vi "Main.vi"(8 "error in (no error)":errorcluster, 11 "GalvoBase in":refnum<class "InVivo_ImagingModeSPIM.lvclass">) -> (0 "error out":errorcluster, 3 "component":refnum<class "InVivo_ImagingModeSPIM.lvclass">)   [LabVIEW 2012, in "InVivo_ImagingModeSPIM.lvclass"]
doc: "Main VI of the component."
uses:
  InVivo_ImagingModeSPIM.lvclass
  <vilib>/Distrio/LabbitMQ/Connection/Connection.lvclass
  <vilib>/Distrio/LabbitMQ/Exchange/Exchange.lvclass
  <vilib>/Distrio/LabbitMQ/Queue/Queue.lvclass
  <vilib>/Distrio/Murmex/TerminateMessage/TerminateMessage.lvclass
  Controls/waveform_enum.ctl
  Control 4.ctl
  InVivo_ImagingModeSPIM.lvclass/InVivo_ImagingModeSPIM.ctl
  <vilib>/Distrio/Murmex/InitialiseMessage/InitialiseMessage.lvclass
  <vilib>/Distrio/Murmex/ConfigureMessage/ConfigureMessage.lvclass
  <vilib>/Distrio/Murmex/StopMessage/StopMessage.lvclass
  <vilib>/Distrio/Murmex/StartMessage/run mode enum.ctl
  <vilib>/Distrio/Murmex/StartMessage/StartMessage.lvclass
  <vilib>/Distrio/Murmex/Murmex/update_cluster.ctl
  <vilib>/Distrio/Murmex/Murmex/Set configure at initialise.vi
  <vilib>/Distrio/Murmex/Murmex/Set VI reference.vi
  <vilib>/Distrio/Murmex/Murmex/Get ID.vi
  <vilib>/Distrio/Murmex/Murmex/Set relay start stop to observers.vi
  <vilib>/Distrio/Murmex/Murmex/Set log reference.vi
  <vilib>/Distrio/Murmex/Murmex/Set license required.vi
  <vilib>/Distrio/Murmex/StartMessage/Set run mode.vi
  <vilib>/Distrio/Murmex/Murmex/Murmex.lvclass
panel:
  in  "button::quit":bool
  in  "button:start_finite":bool
  in  "button:start_free-run":bool
  in  "button::configure":bool
  in  "Tab Control":T1(tab)=enum."Camera"
  in  "Phase 3":dbl[unit] caption="phase" min=-6.283185307179586 max=6.283185307179586 step=0.0017453292519943296
  in  "Offset 3":dbl[unit] caption="offset" min=-5.0 max=5.0 step=0.01
  in  "Amplitude 3":dbl[unit] caption="amplitude" min=0.0 max=5.0 step=0.01
  in  "Phase 2":dbl[unit]=3.14159 caption="phase" min=-6.283185307179586 max=6.283185307179586 step=0.0017453292519943296
  in  "Offset 2":dbl[unit] caption="offset" min=-5.0 max=5.0 step=0.01
  in  "Amplitude 2":dbl[unit] caption="amplitude" min=0.0 max=5.0 step=0.01
  in  "Phase 1":dbl[unit]=3.14159 caption="phase" min=-6.283185307179586 max=6.283185307179586 step=0.0017453292519943296
  in  "shape":T2=enum."sawtooth"
  in  "Offset 1":dbl[unit] caption="offset" min=-5.0 max=5.0 step=0.01
  in  "Amplitude 1":dbl[unit] caption="amplitude" min=0.0 max=5.0 step=0.01
  in  "Amplitude 4":dbl[unit] caption="amplitude" min=0.0 max=5.0 step=0.01
  in  "Offset 4":dbl[unit] caption="offset" min=-5.0 max=5.0 step=0.01
  in  "Phase 4":dbl[unit] caption="phase" min=-6.283185307179586 max=6.283185307179586 step=0.0017453292519943296
  in  "AOTFwaveform":T3
  in  "frame time":dbl[unit]=1.0
  in  "HSYNC pulses":dbl=2048.0 format="%#_6f"
  in  "digital ratio":dbl(knob)=0.5 min=0.0 max=1.0 step=0.02 scale=0.0..1.0
  in  "pulses per pixel":i32 min=0 max=20 step=2
  out "log":string="\r\n16:45:19.783 24/11/2014: initialise from SPIM to SPIM\r\n16:45:20.308 24/11/2014: inform from DAQmxIO to SPIM\r\n16:45:20.427 24/11/2014: inform from SPIM to SPIM\r\n16:45:20.475 24/11/2014: update from SPIM to SPIM\r\n16:45:20.579 24/11/2014: inspect from SPIM to SPIM\r\n16:45:20.660 24/11/2014: inform from SPIM to SPIM\r\n16:45:23.740 24/11/2014: update from SPIM to SPIM\r\n16:45:23.747 24/11/2014: inspect from SPIM to SPIM\r\n16:45:23.824 24/11/2014: inform from SPIM to SPIM\r\n16:45:23.956 24/11/2014: update from SPIM to SPIM\r\n16:45:23.962 24/11/2014: inspect from SPIM to SPIM\r\n16:45:24.038 24/11/2014: inform from SPIM to SPIM\r\n16:45:25.804 24/11/2014: update from SPIM to SPIM\r\n16:45:25.810 24/11/2014: inspect from SPIM to SPIM\r\n16:45:25.891 24/11/2014: inform from SPIM to SPIM\r\n16:45:26.005 24/11/2014: update from SPIM to SPIM\r\n16:45:26.012 24/11/2014: inspect from SPIM to SPIM\r\n16:45:26.088 24/11/2014: inform from SPIM to SPIM\r\n16:45:26.428 24/11/2014: update from SPIM to SPIM\r\n16:45:26.434 24/11/2014: inspect from SPIM to SPIM\r\n16:45:26.514 24/11/2014: inform from SPIM to SPIM\r\n16:45:26.620 24/11/2014: update from SPIM to SPIM\r\n16:45:26.626 24/11/2014: inspect from SPIM to SPIM\r\n16:45:26.703 24/11/2014: inform from SPIM to SPIM\r\n16:45:27.100 24/11/2014: update from SPIM to SPIM\r\n16:45:27.108 24/11/2014: inspect from SPIM to SPIM\r\n16:45:27.184 24/11/2014: inform from SPIM to SPIM\r\n16:45:27.292 24/11/2014: update from SPIM to SPIM\r\n16:45:27.298 24/11/2014: inspect from SPIM to SPIM\r\n16:45:27.380 24/11/2014: inform from SPIM to SPIM\r\n16:45:27.660 24/11/2014: update from SPIM to SPIM\r\n16:45:27.666 24/11/2014: inspect from SPIM to SPIM\r\n16:45:27.743 24/11/2014: inform from SPIM to SPIM\r\n16:45:27.852 24/11/2014: update from SPIM to SPIM\r\n16:45:27.858 24/11/2014: inspect from SPIM to SPIM\r\n16:45:27.934 24/11/2014: inform from SPIM to SPIM\r\n16:45:28.332 24/11/2014: update from SPIM to SPIM\r\n16:45:28.338 24/11/2014: inspect from SPIM to SPIM\r\n16:45:28.421 24/11/2014: inform from SPIM to SPIM\r\n16:45:30.144 24/11/2014: update from SPIM to SPIM\r\n16:45:30.150 24/11/2014: inspect from SPIM to SPIM\r\n16:45:30.232 24/11/2014: inform from SPIM to SPIM\r\n16:45:34.417 24/11/2014: terminate from SPIM to SPIM"
  in  "ID":string="SPIM"
  out "terminate?":bool=TRUE
  # "galvo 1"
  # "galvo 2"
  # "galvo 3"
  # "AOTF"
  # "ImagingModeSPIM\n\nDeveloped by:\n\nMarcel van 't Hoff PhD, \nMarie Caroline Muellenbroich PhD, \nLudovico Silvestri PhD,\n   University of Florence, 2014"
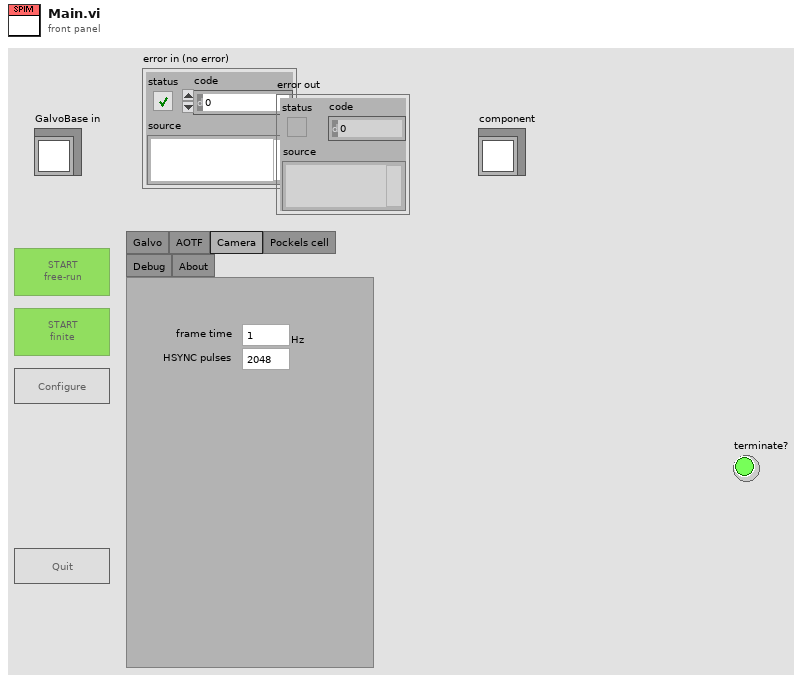
[diagram p1: front panel]
types:
  T1 = enum32{"Galvo", "AOTF", "Camera", "Pockels cell", "Debug", "About"}
  T2 = typedef "InVivo_ImagingModeSPIM.lvclass/waveform_enum.ctl" = enum16{"triangular", "sawtooth", "sinusodial"}
  T3 = typedef "InVivo_ImagingModeSPIM.lvclass/Control 4.ctl" = enum16{"Triangular", "Sawtooth", "Sinusoidal"}
  T4 = enum8{"Enabled", "Disabled", "Disabled and Grayed Out"}
  T5 = typedef "Murmex.lvlib/StartMessage.lvclass/run mode enum.ctl" = enum16{"infinite", "finite"}
  T6 = typedef "Murmex.lvlib/Murmex.lvclass/update_cluster.ctl" = cluster{"target ID":string, "key chains":string[], "values":variant[]}
  T7 = typedef "Murmex.lvlib/Murmex.lvclass/command_enum.ctl" = enum16{"null", "initialise", "reset", "terminate", "acknowledge", "update", "inspect", "inform", "proceed", "start", "stop", "fetch", "configure", "generic"}
  T8 = typedef "Murmex.lvlib/Murmex.lvclass/Event type enumerations.ctl" = enum16{"before", "after"}
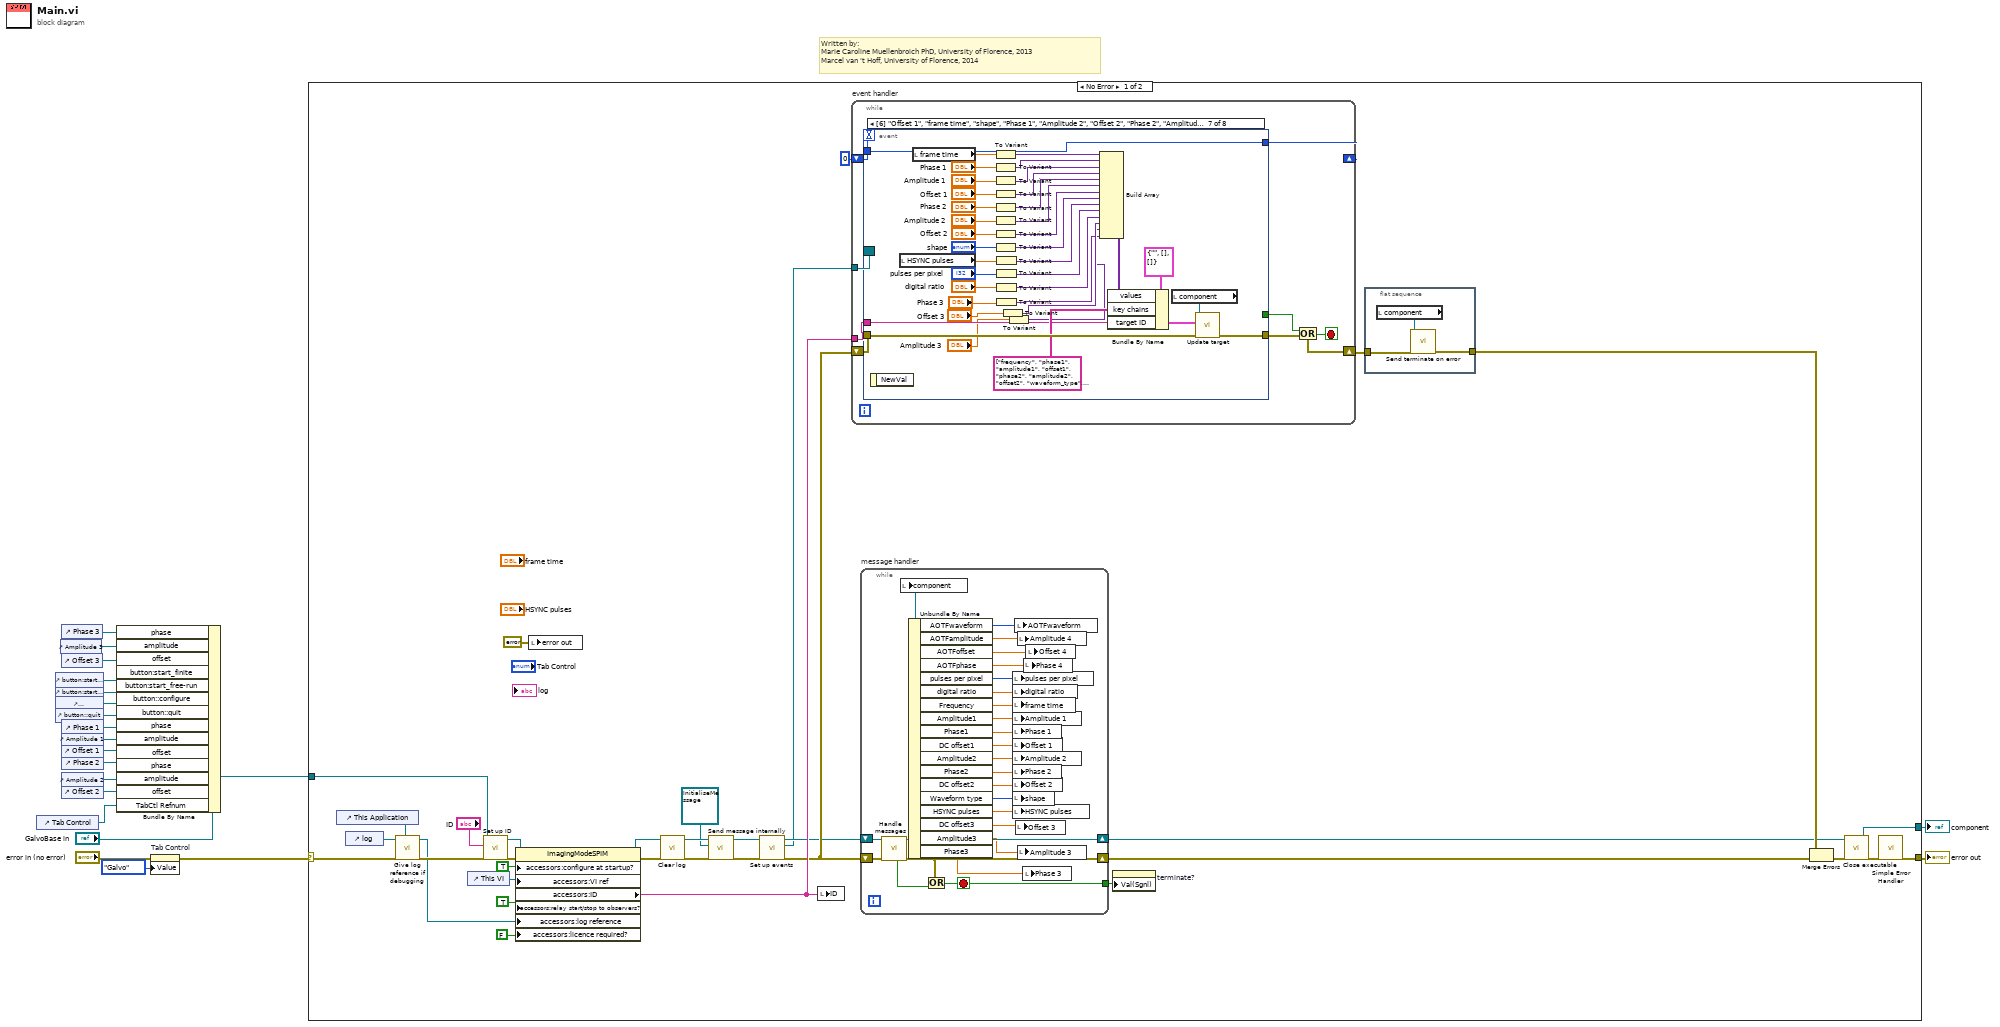
[diagram p0: block diagram]
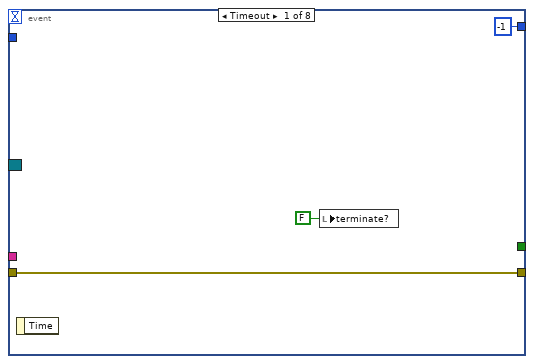
[diagram p2: hidden frame]
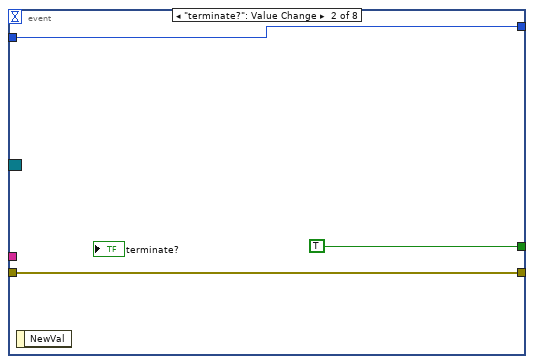
[diagram p3: hidden frame]
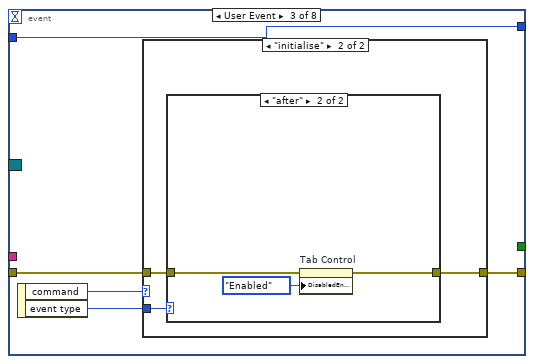
[diagram p4: hidden frame]
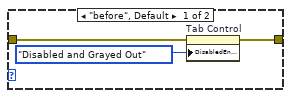
[diagram p6: hidden frame]
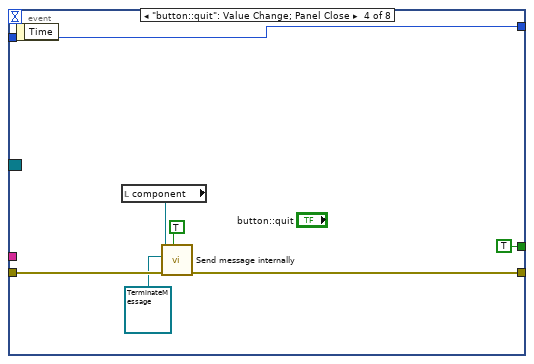
[diagram p7: hidden frame]
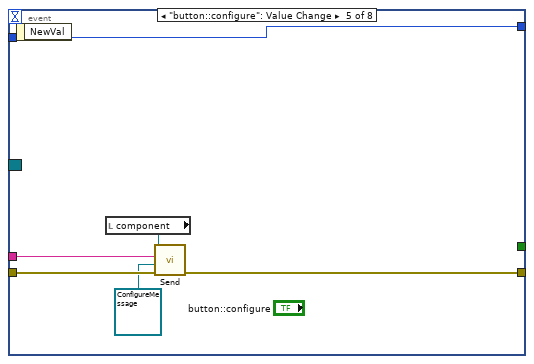
[diagram p8: hidden frame]
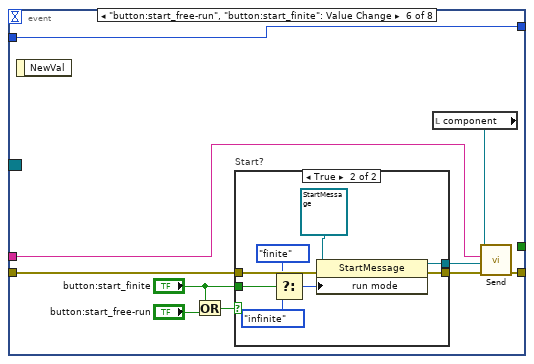
[diagram p9: hidden frame]
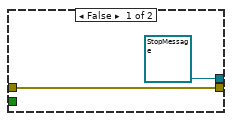
[diagram p10: hidden frame]
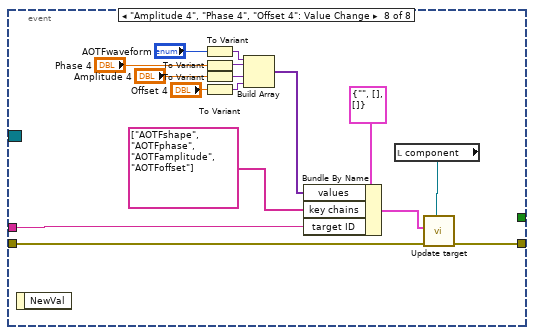
[diagram p11: hidden frame]
diagram:
  # "Written by:\nMarie Caroline Muellenbroich PhD, University of Florence, 2013 \nMarcel van 't Hoff, University of Florence, 2014"
  n1 = control-ref of="Tab Control"() -> (w1:refnum<vi>)
  n2 = control-ref of="button:start_finite"() -> (w18:refnum<vi>)
  n3 = control-ref of="button:start_free-run"() -> (w15:refnum<vi>)
  n4 = control-ref of="button::configure"() -> (w16:refnum<vi>)
  n5 = control-ref of="button::quit"() -> (w17:refnum<vi>)
  n6 = control-ref of="Amplitude 3"() -> (w4:refnum<vi>)
  n7 = control-ref of="Phase 3"() -> (w5:refnum<vi>)
  n8 = control-ref of="Offset 3"() -> (w3:refnum<vi>)
  n9 = control-ref of="Phase 1"() -> (w14:refnum<vi>)
  n10 = control-ref of="Amplitude 1"() -> (w13:refnum<vi>)
  n11 = control-ref of="Offset 1"() -> (w12:refnum<vi>)
  n12 = control-ref of="Phase 2"() -> (w11:refnum<vi>)
  n13 = control-ref of="Amplitude 2"() -> (w10:refnum<vi>)
  n14 = control-ref of="Offset 2"() -> (w9:refnum<vi>)
  n15 = Bundle By Name(cluster="GalvoBase in", "phase"=w5, "amplitude"=w4, "offset"=w3, "button:start_finite"=w18, "button:start_free-run"=w15, "button::configure"=w16, "button::quit"=w17, "phase"=w14, "amplitude"=w13, "offset"=w12, "phase"=w11, "amplitude"=w10, "offset"=w9, "TabCtl Refnum"=w1) -> (w19:refnum<class "InVivo_ImagingModeSPIM.lvclass">)
  n16 = property on="Tab Control" class="TabCtl (strict)"(error in="error in (no error)", "Value"=T1."Galvo" ("Tab Control")) -> (error out=w6:errorcluster)  [unwired: 1 in, 1 out]
  n17 = case shown="No Error" w6 {
    selector: w6 -> [w26 w199]
    tunnel: [w56 w199] -> w21
    tunnel: w19 -> [w38 w200]
    tunnel: [w55 w200] -> w7
    frame No Error {
      n18 = control-ref of="This Application"() -> (w22:refnum<vi>)
      n19 = control-ref of="log"() -> (w24:refnum<vi>)
      n20 = call "Give log reference if debugging.vi"("application ref"=w22, "error in (no error)"=w26, "log reference in"=w24) -> ("error out"=w25:errorcluster, "log reference out"=w23:refnum<vi>)  [unwired: 6 in, 1 out]
      n21 = control-ref of="This VI"() -> (w53:refnum<vi>)
      n22 = call <vilib>:"Set up ID.vi"("error in (no error)"=w25, "component ID"="ID", "MurmexBase in"=w38) -> ("error out"=w50:errorcluster, "MurmexBase out"=w51:refnum<class "InVivo_ImagingModeSPIM.lvclass">)  [unwired: 6 in, 1 out]
      n23 = property class="ImagingModeSPIM"(reference=w51, error in=w50, "accessors:configure at startup?"=TRUE ("configure at startup?"), "accessors:VI ref"=w53, "accessors:relay start/stop to observers?"=TRUE ("relay start/stop to observers?"), "accessors:log reference"=w23, "accessors:licence required?"=FALSE ("licence required?")) -> (reference out=w35:refnum<class "InVivo_ImagingModeSPIM.lvclass">, error out=w37:errorcluster, "accessors:ID"=w40:string)
      n24 = local write "error out"(errorcluster {"status"=FALSE, "code"=0, "source"=""} ("error out")) -> ()
      n25 = call <vilib>:"Clear log.vi"("error in (no error)"=w37, "MurmexBase in"=w35) -> ("error out"=w36:errorcluster, "MurmexBase out"=w34:refnum<class "InVivo_ImagingModeSPIM.lvclass">)  [unwired: 8 in]
      n26 = call <vilib>:"Send message internally.vi"("error in (no error)"=w36, "Message"=refnum<class "InitialiseMessage.lvclass"> refnum ("Murmex.lvlib:InitialiseMessage"), "Murmex in"=w34) -> ("error out"=w31:errorcluster, "Murmex out"=w29:refnum<class "InVivo_ImagingModeSPIM.lvclass">)  [unwired: 7 in]
      n27 = call <vilib>:"Set up events.vi"("error in (no error)"=w31, "MurmexBase in"=w29) -> ("error out"=w30:errorcluster, "Event Registration Refnum"=w27:refnum<event-registration>, "MurmexBase out"=w28:refnum<class "InVivo_ImagingModeSPIM.lvclass">)  [unwired: 7 in]
      n28 = local write "ID"(w40) -> ()
      n29 = while "event handler" {
        shift-right: [w65] -> w48
        shift-left: w30 -> [w67]
        shift-right: [w61] -> _
        shift-left: 0 -> [w62]
        tunnel: w40 -> [w63]
        tunnel: w27 -> [w60]
        stop <- w64 stop-if-true
        n30 = event shown="[6] \"Offset 1\", \"frame time\", \"shape\", \"Phase 1\", \"Amplitude 2\", \"Offset 2\", \"Phase 2\", \"Amplitude 1\", \"HSYNC pulses\", \"pulses per pixel\", \"digital ratio\", \"Offset 3\", \"Phase 3\", \"Amplitude 3\": Value Change" {
          selector: w60 -> [_ _ _ _ _ _ _ _]
          dyn-events: _ -> [_ _ _ _ _ _ _ _]
          timeout: w62 -> [_ _ _ _ _ _ _ _]
          tunnel: [w70 w73 w75 w95 w100 w105 w157 w165] -> w65
          tunnel: w67 -> [w70 w73 w76 w94 w101 w110 w158 w166]
          tunnel: [_ TRUE ("configure at startup?") _ TRUE ("configure at startup?") _ _ _ _] -> w66
          tunnel: w63 -> [_ _ _ _ w99 w102 w136 w170]
          tunnel: w62 -> [_ w71 w74 w92 w98 w111 w144 _]
          tunnel: [-1 w71 w74 w92 w98 w111 w144 _] -> w61
          event Timeout {
            n31 = event-data() -> ()  [unwired: 1 in, 1 out]
            n32 = local write "terminate?"(FALSE ("terminate?")) -> ()
          }
          event "terminate?": Value Change {
            n33 = event-data() -> ()  [unwired: 1 in, 1 out]
          }
          event User Event {
            n34 = event-data() -> ("command"=w78:T7, "event type"=w77:T8)  [unwired: 1 in]
            n35 = case shown="\"initialise\"" w78 {
              tunnel: w77 -> [_ w82]
              tunnel: w76 -> [w79 w81]
              tunnel: [w79 w80] -> w75
              frame "null", Default {
              }
              frame "initialise" {
                n36 = case shown="\"after\"" w82 {
                  tunnel: w81 -> [w85 w88]
                  tunnel: [w84 w87] -> w80
                  frame "before", Default {
                    n37 = property on="Tab Control" class="TabCtl (strict)"(error in=w85, "DisabledEnum"=T4."Disabled and Grayed Out" ("Disabled")) -> (error out=w84:errorcluster)  [unwired: 1 in, 1 out]
                  }
                  frame "after" {
                    n38 = property on="Tab Control" class="TabCtl (strict)"(error in=w88, "DisabledEnum"=T4."Enabled" ("Disabled")) -> (error out=w87:errorcluster)  [unwired: 1 in, 1 out]
                  }
                }
              }
            }
          }
          event "button::quit": Value Change; Panel Close {
            n39 = event-data() -> ()  [unwired: 1 in, 1 out]
            n40 = local read "component"() -> (w91:refnum<class "InVivo_ImagingModeSPIM.lvclass">)
            n41 = call <vilib>:"Send message internally.vi"("priority message? (F)"=TRUE, "error in (no error)"=w94, "Message"=refnum<class "TerminateMessage.lvclass"> refnum ("Murmex.lvlib:TerminateMessage"), "Murmex in"=w91) -> ("error out"=w95:errorcluster)  [unwired: 6 in, 1 out]
          }
          event "button::configure": Value Change {
            n42 = event-data() -> ()  [unwired: 1 in, 1 out]
            n43 = local read "component"() -> (w97:refnum<class "InVivo_ImagingModeSPIM.lvclass">)
            n44 = call <vilib>:"Send.vi"("error in (no error)"=w101, "Message"=refnum<class "ConfigureMessage.lvclass"> refnum ("Murmex.lvlib:ConfigureMessage"), "recipient"=w99, "Murmex in"=w97) -> ("error out"=w100:errorcluster)  [unwired: 6 in, 1 out]
          }
          event "button:start_free-run", "button:start_finite": Value Change {
            n45 = event-data() -> ()  [unwired: 1 in, 1 out]
            n46 = Or(x="button:start_finite", y="button:start_free-run") -> (x .or. y?=w109:bool)
            n47 = case "Start?" shown="True" w109 {
              tunnel: w110 -> [w113 w121]
              tunnel: [w113 w116] -> w106
              tunnel: "button:start_finite" -> [_ w117]
              tunnel: [refnum<class "StopMessage.lvclass"> refnum ("Murmex.lvlib:StopMessage") w115] -> w103
              frame False {
              }
              frame True {
                n48 = Select(t=run_mode_enum."finite" ("run mode"), s=w117, f=run_mode_enum."infinite" ("run mode")) -> (s? t:f=w118:T5)
                n49 = property class="StartMessage"(reference=refnum<class "StartMessage.lvclass"> refnum ("Murmex.lvlib:StartMessage"), error in=w121, "run mode"=w118) -> (reference out=w115:refnum<class "StartMessage.lvclass">, error out=w116:errorcluster)
              }
            }
            n50 = local read "component"() -> (w104:refnum<class "InVivo_ImagingModeSPIM.lvclass">)
            n51 = call <vilib>:"Send.vi"("error in (no error)"=w106, "Message"=w103, "recipient"=w102, "Murmex in"=w104) -> ("error out"=w105:errorcluster)  [unwired: 6 in, 1 out]
          }
          event "Offset 1", "frame time", "Phase 1", "Amplitude 2", "Offset 2", "Phase 2", "Amplitude 1", "HSYNC pulses", "pulses per pixel", "digital ratio", "Offset 3", "Phase 3", "Amplitude 3": Value Change {
            n52 = event-data() -> ()  [unwired: 1 in, 1 out]
            n53 = local read "HSYNC pulses"() -> (w129:dbl)
            n54 = local read "frame time"() -> (w128:dbl[unit])
            n55 = To Variant(anything=w128) -> (Variant=w154:variant)
            n56 = To Variant(anything="Phase 1") -> (Variant=w151:variant)
            n57 = To Variant(anything="Amplitude 1") -> (Variant=w150:variant)
            n58 = To Variant(anything="Offset 1") -> (Variant=w149:variant)
            n59 = To Variant(anything="Phase 2") -> (Variant=w141:variant)
            n60 = To Variant(anything="Amplitude 2") -> (Variant=w140:variant)
            n61 = To Variant(anything="Offset 2") -> (Variant=w137:variant)
            n62 = To Variant(anything="shape") -> (Variant=w143:variant)
            n63 = To Variant(anything=w129) -> (Variant=w134:variant)
            n64 = To Variant(anything="pulses per pixel") -> (Variant=w132:variant)
            n65 = To Variant(anything="digital ratio") -> (Variant=w131:variant)
            n66 = To Variant(anything="Phase 3") -> (Variant=w122:variant)
            n67 = To Variant(anything="Offset 3") -> (Variant=w124:variant)
            n68 = To Variant(anything="Amplitude 3") -> (Variant=w123:variant)
            n69 = Build Array(w154, w151, w150, w149, w141, w140, w137, w143, w134, w132, w131, w124, w123, w122) -> (w153:variant[])
            n70 = Bundle By Name(cluster=T6 {"target ID"="", "key chains"=[], "values"=[]} ("update cluster"), "values"=w153, "key chains"=string[] ["frequency", "phase1", "amplitude1", "offset1", "phase2", "amplitude2", "offset2", "waveform_type", "hsync_pulses", "pulses_per_pixel", "digital_ratio", "offset3", "amplitude3", "phase3"], "target ID"=w136) -> (w155:T6)
            n71 = local read "component"() -> (w135:refnum<class "InVivo_ImagingModeSPIM.lvclass">)
            n72 = call <vilib>:"Update target.vi"("error in (no error)"=w158, "update cluster"=w155, "MurmexBase in"=w135) -> ("error out"=w157:errorcluster)  [unwired: 7 in, 1 out]
          }
          event "Amplitude 4", "Phase 4", "Offset 4": Value Change {
            n73 = event-data() -> ()  [unwired: 1 in, 1 out]
            n74 = To Variant(anything="AOTFwaveform") -> (Variant=w160:variant)
            n75 = To Variant(anything="Phase 4") -> (Variant=w172:variant)
            n76 = To Variant(anything="Amplitude 4") -> (Variant=w173:variant)
            n77 = To Variant(anything="Offset 4") -> (Variant=w174:variant)
            n78 = Build Array(w160, w172, w173, w174) -> (w171:variant[])
            n79 = Bundle By Name(cluster=T6 {"target ID"="", "key chains"=[], "values"=[]} ("update cluster"), "values"=w171, "key chains"=string[] ["AOTFshape", "AOTFphase", "AOTFamplitude", "AOTFoffset"], "target ID"=w170) -> (w167:T6)
            n80 = local read "component"() -> (w164:refnum<class "InVivo_ImagingModeSPIM.lvclass">)
            n81 = call <vilib>:"Update target.vi"("error in (no error)"=w166, "update cluster"=w167, "MurmexBase in"=w164) -> ("error out"=w165:errorcluster)  [unwired: 7 in, 1 out]
          }
        }
        n82 = Or(x=w66, y=w65) -> (x .or. y?=w64:bool)
      }
      n83 = while "message handler" {
        shift-right: [w183] -> w43
        shift-left: w28 -> [w197]
        shift-right: [w196] -> w46
        shift-left: w30 -> [w198]
        tunnel: [w194] -> w52
        stop <- w194 stop-if-true
        n84 = call <vilib>:"Handle messages.vi"("error in (no error)"=w198, "Murmex in"=w197) -> ("error out"=w196:errorcluster, "Murmex out"=w183:refnum<class "InVivo_ImagingModeSPIM.lvclass">, "terminated?"=w195:bool)  [unwired: 7 in]
        n85 = local write "component"(w183) -> ()
        n86 = Unbundle By Name(w183) -> ("AOTFwaveform"=w175:T3, "AOTFamplitude"=w178:dbl[unit], "AOTFoffset"=w176:dbl[unit], "AOTFphase"=w177:dbl[unit], "pulses per pixel"=w184:i32, "digital ratio"=w185:dbl, "Frequency"=w182:dbl[unit], "Amplitude1"=w193:dbl[unit], "Phase1"=w191:dbl[unit], "DC offset1"=w189:dbl[unit], "Amplitude2"=w192:dbl[unit], "Phase2"=w190:dbl[unit], "DC offset2"=w188:dbl[unit], "Waveform type"=w187:T2, "HSYNC pulses"=w186:dbl, "DC offset3"=w181:dbl[unit], "Amplitude3"=w180:dbl[unit], "Phase3"=w179:dbl[unit])
        n87 = Or(x=w196, y=w195) -> (x .or. y?=w194:bool)
        n88 = local write "pulses per pixel"(w184) -> ()
        n89 = local write "digital ratio"(w185) -> ()
        n90 = local write "frame time"(w182) -> ()
        n91 = local write "Amplitude 1"(w193) -> ()
        n92 = local write "Phase 1"(w191) -> ()
        n93 = local write "Offset 1"(w189) -> ()
        n94 = local write "Amplitude 2"(w192) -> ()
        n95 = local write "Phase 2"(w190) -> ()
        n96 = local write "Offset 2"(w188) -> ()
        n97 = local write "shape"(w187) -> ()
        n98 = local write "HSYNC pulses"(w186) -> ()
        n99 = local write "AOTFwaveform"(w175) -> ()
        n100 = local write "Offset 3"(w181) -> ()
        n101 = local write "Amplitude 4"(w178) -> ()
        n102 = local write "Amplitude 3"(w180) -> ()
        n103 = local write "Phase 3"(w179) -> ()
        n104 = local write "Phase 4"(w177) -> ()
        n105 = local write "Offset 4"(w176) -> ()
      }
      n106 = property on="terminate?" class="Bool (strict)"("Val(Sgnl)"=w52) -> ()  [unwired: 2 in, 2 out]
      n107 = flat-sequence {
        tunnel: w48 -> [w59]
        tunnel: [w57] -> w47
        frame #0 {
          n108 = local read "component"() -> (w58:refnum<class "InVivo_ImagingModeSPIM.lvclass">)
          n109 = call <vilib>:"Send terminate on error.vi"("error in (no error)"=w59, "Murmex in"=w58) -> ("error out"=w57:errorcluster)  [unwired: 8 in, 1 out]
        }
      }
      n110 = Merge Errors(w47, w46) -> (w45:errorcluster)
      n111 = call <vilib>:"Close executable.vi"("error in (no error)"=w45, "MurmexBase in"=w43) -> ("error out"=w44:errorcluster, "MurmexBase out"=w55:refnum<class "InVivo_ImagingModeSPIM.lvclass">)  [unwired: 8 in]
      n112 = call <vilib>:"Simple Error Handler.vi"("error in (no error)"=w44) -> ("error out"=w56:errorcluster)  [unwired: 4 in, 4 out]
    }
    frame Error {
    }
  }
  "error out" <- w21
  "component" <- w7
